vi "FT_Set_Data_Characteristics.vi"(1 "Parity":u8(ring) items=["FT_PARITY_NONE", "FT_PARITY_ODD", "FT_PARITY_EVEN", "FT_PARITY_MARK", "FT_PARITY_SPACE"], 2 "Stop Bits":u8(ring) items=["FT_STOP_BITS_1"=0, "FT_STOP_BITS_2"=2], 3 "Word Length":u8(ring)=8 items=["FT_BITS_7"=7, "FT_BITS_8"=8], 4 "Handle":u32) -> (0 "FT_Status":u32(ring) items=["FT_OK", "FT_INVALID_HANDLE", "FT_DEVICE_NOT_FOUND", "FT_DEVICE_NOT_OPENED", "FT_IO_ERROR", "FT_INSUFFICIENT_RESOURCES", "FT_INVALID_PARAMETER", "FT_INVALID_BAUD_RATE", "FT_DEVICE_NOT_OPENED_FOR_ERASE", "FT_DEVICE_NOT_OPENED_FOR_WRITE", "FT_FAILED_TO_WRITE_DEVICE", "FT_EEPROM_READ_FAILED", "FT_EEPROM_WRITE_FAILED", "FT_EEPROM_ERASE_FAILED", "FT_EEPROM_NOT_PRESENT", "FT_EEPROM_NOT_PROGRAMMED", "FT_INVALID_ARGS", "FT_NOT_SUPPORTED", "FT_OTHER_ERROR"])   [LabVIEW 2011]
uses:
  ftd2xx.dll
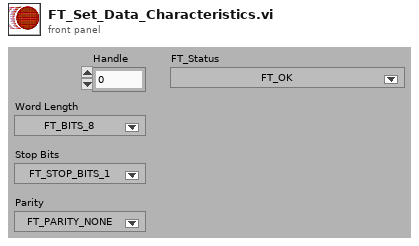
[diagram p1: front panel]
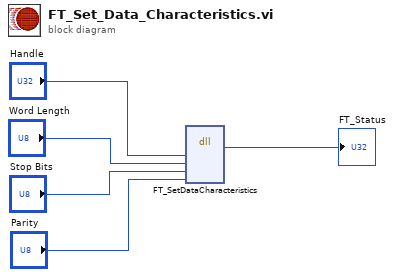
[diagram p0: block diagram]
diagram:
  n1 = dll-call lib="C:/Users/INL Students/Desktop/INL labview repository/3rd Party/D2XX_Functions_7.0/FTD2XX.dll" fn="FT_SetDataCharacteristics" label="FT_SetDataCharactceristics"("Handle"="Handle", "WordLength"="Word Length", "StopBits"="Stop Bits", "Parity"="Parity") -> ("FT_Status"=→"FT_Status":u32)  [unwired: 7 in, 2 out]
